vi "Configure Trigger.vi"(8 "error in (no error)":errorcluster, 9 "trigger delay (0.0 s)":dbl format="%.3f", 10 "trigger source (Immediate)":i32(ring)=1 items=["Immediate"=1, "External"=2, "Software Trigger Function"=3, "PXI TRIG0 or VXI TTL0"=111, "PXI TRIG1 or VXI TTL1"=112, "PXI TRIG2 or VXI TTL2"=113, "PXI TRIG3 or VXI TTL3"=114, "PXI TRIG4 or VXI TTL4"=115, "PXI TRIG5 or VXI TTL5"=116, "PXI TRIG6 or VXI TTL6"=117, "PXI TRIG7 or VXI TTL7"=118, "ECL0"=119, "ECL1"=120, "PXI Star"=131, "RTSI 0"=140, "RTSI 1"=141, "RTSI 2"=142, "RTSI 3"=143, "RTSI 4"=144, "RTSI 5"=145, "RTSI 6"=146], 11 "CS++DMM in":refnum<class "CS++DMM.lvclass">) -> (0 "error out":errorcluster, 3 "CS++DMM out":refnum<class "CS++DMM.lvclass">)   [LabVIEW 2013, in "CS++DMM.lvlib" / "CS++DMM.lvclass"]
doc: "This VI configures the common DMM trigger properties. These properties are the trigger source and trigger delay."
uses:
  CS++DMM.lvclass
  CSPP_Core/Classes/CS++ProcessVariables/ProcessVariable/PV.lvclass
  CSPP_Core/Classes/CS++ProcessVariables/ProcessVariable/PV.lvclass/PV.ctl
  CS++DMM.lvclass/CS++DMM.ctl
  CSPP_Core/Classes/CS++ProcessVariables/PVConnection/PVConnection.lvclass
  CSPP_Core/Classes/CS++ProcessVariables/ProcessVariable/Write Data.vi
  CSPP_Core/Classes/CS++ProcessVariables/ProcessVariable/Write Timestamp.vi
  CSPP_Core/Classes/CS++ProcessVariables/ProcessVariable/Write Quality.vi
  CSPP_Core/Classes/CS++ProcessVariables/ProcessVariable/Write status.vi
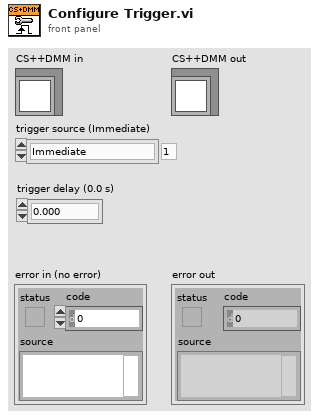
[diagram p1: front panel]
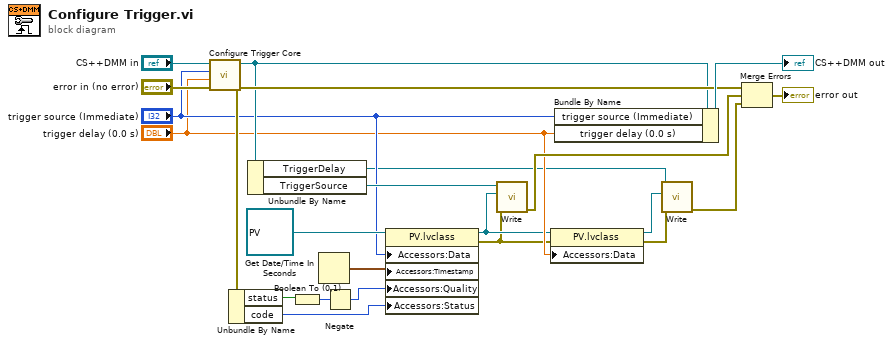
[diagram p0: block diagram]
diagram:
  n1 = call-dynamic "Configure Trigger Core.vi"("error in (no error)"="error in (no error)", "trigger delay (0.0 s)"="trigger delay (0.0 s)", "trigger source (Immediate)"="trigger source (Immediate)", "CS++DMM in"="CS++DMM in") -> ("error out"=w11:errorcluster, "CS++DMM out"=w10:refnum<class "CS++DMM.lvclass">)  [unwired: 6 in]
  n2 = Unbundle By Name(w11) -> ("status"=w17:bool, "code"=w14:i32)
  n3 = Unbundle By Name(w10) -> ("TriggerDelay"=w1:refnum<class "PVConnection.lvclass">, "TriggerSource"=w12:refnum<class "PVConnection.lvclass">)
  n4 = Boolean To (0,1)(Boolean=w17) -> (0, 1=w16:i16)
  n5 = Get Date/Time In Seconds() -> (seconds since 1Jan1904=w13:timestamp)
  n6 = Negate(x=w16) -> (-x=w15:i16)
  n7 = property class="PV.lvclass"(reference=refnum<class "PV.lvclass"> refnum ("CS++ProcessVariables.lvlib:PV.lvclass"), "Accessors:Data"="trigger source (Immediate)", "Accessors:Timestamp"=w13, "Accessors:Quality"=w15, "Accessors:Status"=w14) -> (reference out=w4:refnum<class "PV.lvclass">, error out=w3:errorcluster)  [unwired: 1 in]
  n8 = call-dynamic "Write.vi"("error in (no error)"=w3, "PV"=w4, "PVConnection in"=w12) -> ("error out"=w8:errorcluster)  [unwired: 7 in, 1 out]
  n9 = property class="PV.lvclass"(reference=w4, error in=w3, "Accessors:Data"="trigger delay (0.0 s)") -> (reference out=w6:refnum<class "PV.lvclass">, error out=w7:errorcluster)
  n10 = Bundle By Name(cluster=w10, "trigger source (Immediate)"="trigger source (Immediate)", "trigger delay (0.0 s)"="trigger delay (0.0 s)") -> (→"CS++DMM out":refnum<class "CS++DMM.lvclass">)
  n11 = call-dynamic "Write.vi"("error in (no error)"=w7, "PV"=w6, "PVConnection in"=w1) -> ("error out"=w2:errorcluster)  [unwired: 7 in, 1 out]
  n12 = Merge Errors(w11, w8, w2) -> (→"error out":errorcluster)
